vi "Logger Daemon.vi"(8 "Error In":errorcluster, 11 "TDMS Log In":refnum<class "TDMS Logger.lvclass">) -> ()   [LabVIEW 2015, in "TDMS Logger.lvlib" / "TDMS Logger.lvclass"]
uses:
  TDMS Logger.lvclass
  TDMS Logger.lvclass/TDMS Logger.ctl
  _Typedefs/Log Message.ctl
  _Typedefs/Log Action.ctl
  _Typedefs/Data Type.ctl
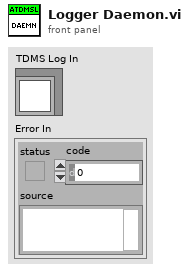
[diagram p1: front panel]
types:
  T1 = typedef "TDMS Logger.lvlib/TDMS Logger.lvclass/Log Action.ctl" = enum16{"Handle Old Files", "Status Update", "Stop", "Log Data", "Initialize"}
  T2 = typedef "TDMS Logger.lvlib/TDMS Logger.lvclass/Log Message.ctl" = cluster{"Log Action":T1, "Variant":variant, "Data Type":T3, "Group Name":string, "Channels Names":string[]}
  T3 = typedef "TDMS Logger.lvlib/TDMS Logger.lvclass/Data Type.ctl" = enum16{"I16", "I8", "String", "U16", "U8", "Waveform", "Double", "Single"}
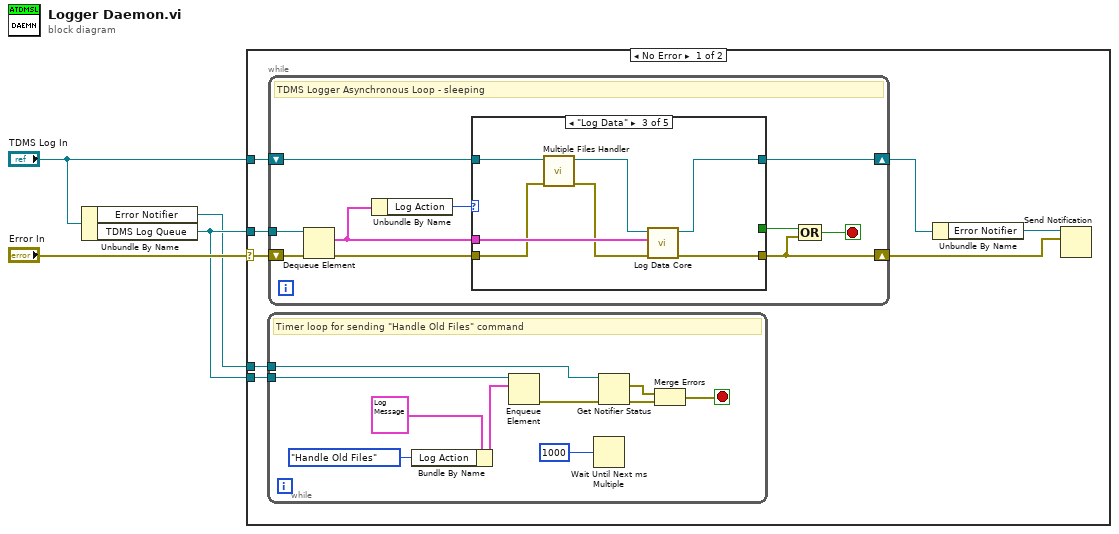
[diagram p0: block diagram]
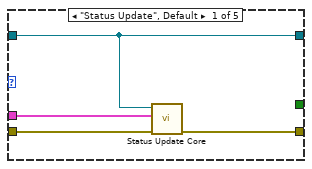
[diagram p2: hidden frame]
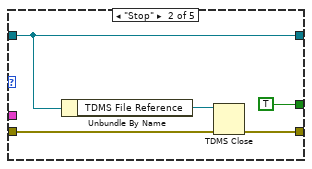
[diagram p3: hidden frame]
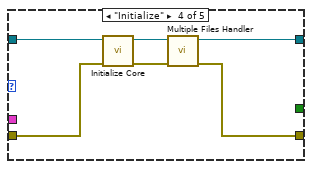
[diagram p4: hidden frame]
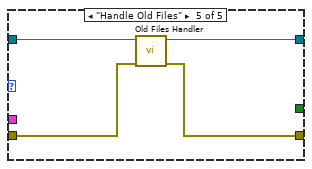
[diagram p5: hidden frame]
diagram:
  n1 = Unbundle By Name("TDMS Log In") -> ("Error Notifier"=w1:refnum<notifier>, "TDMS Log Queue"=w2:refnum<queue>)
  n2 = case shown="No Error" "Error In" {
    selector: "Error In" -> [w11 _]
    tunnel: "TDMS Log In" -> [w12 _]
    tunnel: w2 -> [w10 _]
    tunnel: w2 -> [w6 _]
    tunnel: w1 -> [w5 _]
    frame No Error {
      n3 = while {
        tunnel: w6 -> [w22]
        tunnel: w5 -> [w16]
        stop <- w13 stop-if-true
        # "Timer loop for sending \"Handle Old Files\" command"
        n4 = Bundle By Name(cluster=T2 {"Log Action"=enum."Stop", "Variant"=variant, "Data Type"=enum."String", "Group Name"="", "Channels Names"=[]} ("element"), "Log Action"=Log_Action."Handle Old Files") -> (w18:T2)
        n5 = Enqueue Element(queue=w22, element=w18) -> (error out=w17:errorcluster)  [unwired: 2 in, 2 out]
        n6 = Wait Until Next ms Multiple(millisecond multiple=u32 1000) -> ()  [unwired: 1 out]
        n7 = Get Notifier Status(notifier=w16, error in (no error)=w17) -> (current notification=w14:errorcluster, error out=w15:errorcluster)  [unwired: 3 out]
        n8 = Merge Errors(w14, w15) -> (w13:errorcluster)
      }
      n9 = while {
        shift-right: [w24] -> w9
        shift-left: w12 -> [w26]
        tunnel: w10 -> [w31]
        shift-right: [w23] -> w7
        shift-left: w11 -> [w32]
        stop <- w27 stop-if-true
        # "TDMS Logger Asynchronous Loop - sleeping"
        n10 = Dequeue Element(queue=w31, error in (no error)=w32) -> (element=w29:T2, error out=w25:errorcluster)  [unwired: 1 in, 2 out]
        n11 = Unbundle By Name(w29) -> ("Log Action"=w30:T1)
        n12 = case shown="\"Log Data\"" w30 {
          tunnel: w29 -> [w36 _ w48 _ _]
          tunnel: w25 -> [w34 w40 w46 w49 w56]
          tunnel: [w33 w39 w45 w52 w55] -> w23
          tunnel: [_ TRUE _ _ _] -> w28
          tunnel: [w35 w38 w44 w53 w57] -> w24
          tunnel: w26 -> [w35 w38 w47 w54 w58]
          frame "Status Update", Default {
            n13 = call "Status Update Core.vi"("Error In"=w34, "Log Message"=w36, "TDMS Log In"=w35) -> ("Error Out"=w33:errorcluster)  [unwired: 8 in]
          }
          frame "Stop" {
            n14 = Unbundle By Name(w38) -> ("TDMS File Reference"=w37:refnum<k34>)
            n15 = TDMS Close(8:w40, 11:w37) -> (0:w39:errorcluster)  [unwired: 1 out]
          }
          frame "Log Data" {
            n16 = call "Multiple Files Handler.vi"("Error In"=w46, "TDMS Log"=w47) -> ("Error Out"=w42:errorcluster, "TDMS Log Out"=w43:refnum<class "TDMS Logger.lvclass">)  [unwired: 8 in]
            n17 = call "Log Data Core.vi"("Error In"=w42, "Log Message"=w48, "TDMS Log In"=w43) -> ("Error Out"=w45:errorcluster, "TDMS Log Out"=w44:refnum<class "TDMS Logger.lvclass">)  [unwired: 7 in]
          }
          frame "Initialize" {
            n18 = call "Initialize Core.vi"("Error In"=w49, "TDMS Log In"=w54) -> ("Error Out"=w50:errorcluster, "TDMS Log Out"=w51:refnum<class "TDMS Logger.lvclass">)  [unwired: 8 in]
            n19 = call "Multiple Files Handler.vi"("Error In"=w50, "TDMS Log"=w51) -> ("Error Out"=w52:errorcluster, "TDMS Log Out"=w53:refnum<class "TDMS Logger.lvclass">)  [unwired: 8 in]
          }
          frame "Handle Old Files" {
            n20 = call "Old Files Handler.vi"("Error In"=w56, "TDMS Log"=w58) -> ("Error Out"=w55:errorcluster, "TDMS Log"=w57:refnum<class "TDMS Logger.lvclass">)  [unwired: 8 in]
          }
        }
        n21 = Compound Arithmetic op=OR(w28, w23) -> (w27:bool)
      }
      n22 = Unbundle By Name(w9) -> ("Error Notifier"=w8:refnum<notifier>)
      n23 = Send Notification(notification=w7, notifier=w8) -> ()  [unwired: 1 in, 2 out]
    }
    frame Error {
    }
  }
